vi "Draw Picture Grid.vi"(9 "Draw Area Size":T1, 11 "picture in":picture) -> (3 "picture out":picture)   [LabVIEW 2025]
doc: "Draw reticule, centered grid lines."
uses:
  <vilib>/Utility/miscctls.llb/LVBoundsTypeDef.ctl
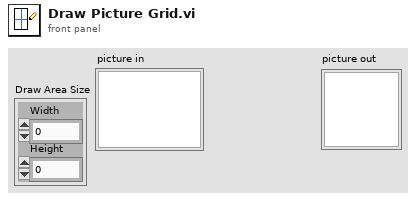
[diagram p1: front panel]
types:
  T1 = typedef "LVBoundsTypeDef.ctl" = cluster{"Width":u32, "Height":u32}
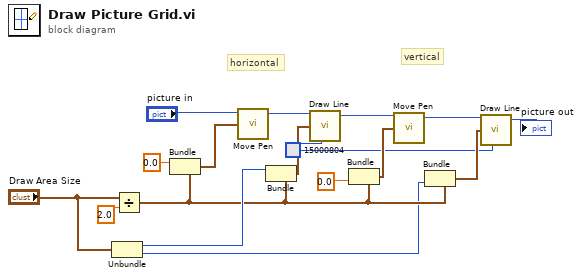
[diagram p0: block diagram]
diagram:
  w1 = u32 15000804 ("color(black)")
  # "vertical"
  # "horizontal"
  n1 = Unbundle("Draw Area Size") -> ("Width"=w7:u32, "Height"=w3:u32)
  n2 = Divide(x="Draw Area Size", y=2.0) -> (x/y=w4:cluster{"Width":dbl, "Height":dbl})
  n3 = Bundle(cluster=w4, "Width"=0.0) -> (w10:cluster{"Width":dbl, "Height":dbl})  [unwired: 1 in]
  n4 = call <vilib>:"Move Pen.vi"("new position"=w10, "picture"="picture in") -> ("new picture"=w14:picture)  [unwired: 3 in]
  n5 = Bundle(cluster=w4, "Width"=w7) -> (w8:cluster{"Width":dbl, "Height":dbl})  [unwired: 1 in]
  n6 = call <vilib>:"Draw Line.vi"("picture"=w14, "end point"=w8, "color(black)"=w1) -> ("new picture"=w13:picture)  [unwired: 6 in]
  n7 = Bundle(cluster=w4, "Height"=0.0 ("Width")) -> (w6:cluster{"Width":dbl, "Height":dbl})  [unwired: 1 in]
  n8 = call <vilib>:"Move Pen.vi"("new position"=w6, "picture"=w13) -> ("new picture"=w12:picture)  [unwired: 3 in]
  n9 = Bundle(cluster=w4, "Height"=w3) -> (w5:cluster{"Width":dbl, "Height":dbl})  [unwired: 1 in]
  n10 = call <vilib>:"Draw Line.vi"("picture"=w12, "end point"=w5, "color(black)"=w1) -> ("new picture"=→"picture out":picture)  [unwired: 6 in]
